vi "Clockwise.vi"(8 "Modbus instance in":refnum<class "Modbus API.lvclass">, 11 "error in":errorcluster) -> (0 "Modbus instance out":refnum<class "Modbus API.lvclass">, 3 "error out":errorcluster)   [LabVIEW 2014, in "Files Library.lvlib"]
uses:
  Files Library.lvlib
  <vilib>/NI/Modbus Library/API/Modbus API.lvclass
  Global/ClockWise Global.vi
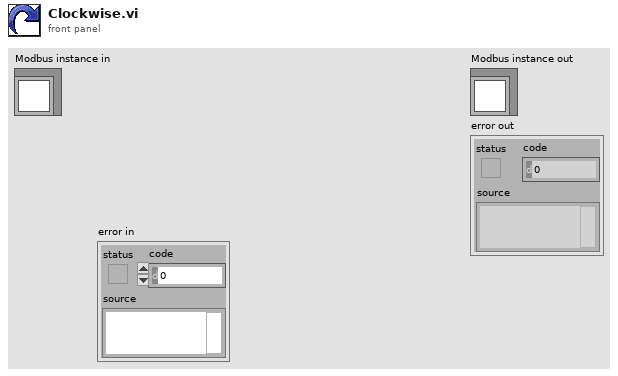
[diagram p1: front panel]
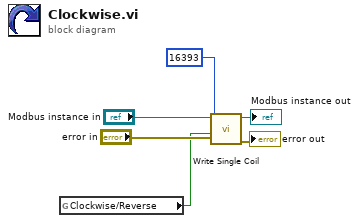
[diagram p0: block diagram]
diagram:
  n1 = global read "ClockWise Global.vi" "Clockwise/Reverse"() -> (w1:bool)
  n2 = call-dynamic "Write Single Coil.vi"("error in"="error in", "coil to write"=w1, "address"=u16 16393, "Modbus instance in"="Modbus instance in") -> ("error out"=→"error out":errorcluster, "Modbus instance out"=→"Modbus instance out":refnum<class "Modbus API.lvclass">)  [unwired: 6 in]
